vi "Read previous state.vi"(8 "error in (no error)":errorcluster, 11 "StateManager in":refnum<class "StateManager.lvclass">) -> (0 "error out":errorcluster, 2 "previousState":u32, 3 "StateManager out":refnum<class "StateManager.lvclass">)   [LabVIEW 2018, in "StateManager.lvclass"]
uses:
  StateManager.lvclass
  StateManager.lvclass/StateManager.ctl
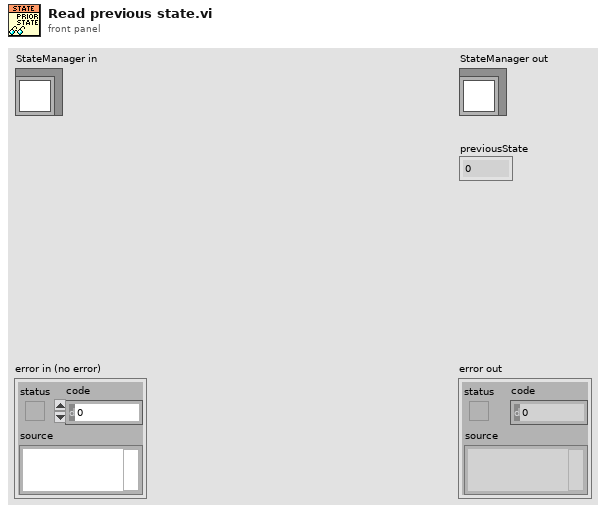
[diagram p1: front panel]
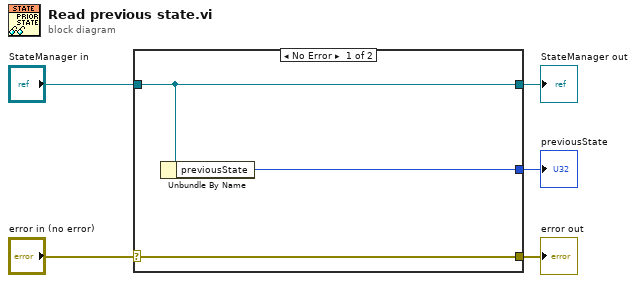
[diagram p0: block diagram]
diagram:
  n1 = case shown="No Error" "error in (no error)" {
    selector: "error in (no error)" -> [w8 w9]
    tunnel: [w8 w9] -> w4
    tunnel: [w7 w10] -> w2
    tunnel: "StateManager in" -> [w7 w10]
    tunnel: [w6 _] -> w1
    frame No Error {
      n2 = Unbundle By Name(w7) -> ("previousState"=w6:u32)
    }
    frame Error {
    }
  }
  "error out" <- w4
  "StateManager out" <- w2
  "previousState" <- w1
